vi "Build Bank Engine Group.vi"(8 "error in (no error)":errorcluster, 11 "Device ref dup":T1 format="%.0x") -> (0 "error out":errorcluster, 2 "Group":T2 {"VS Refs" format="%.0x"}, 3 "Section Ref out":T1 format="%.0x")   [LabVIEW 2017, in "NI 272x Resistive Simulation Custom Device Configuration.lvlib"]
uses:
  NI 272x Resistive Simulation Custom Device Configuration.lvlib
  <vilib>/NI Veristand/Custom Device API/Custom Device Item Ref.ctl
  <vilib>/NI Veristand/Custom Device Tools/Custom Device Utility Library/NI VeriStand - Search for Item by Name.vi
  <vilib>/NI VeriStand/Custom Device Tools/Custom Device Utility Library/Custom Device Utility Library.lvlib
  <vilib>/NI VeriStand/Custom Device API/Custom Device API.lvlib
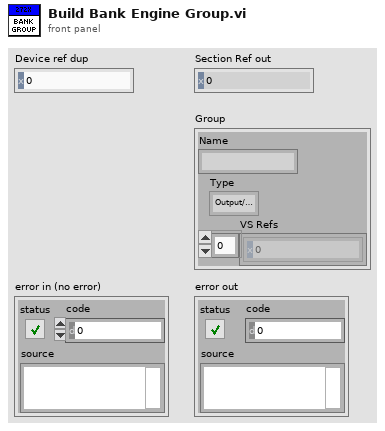
[diagram p1: front panel]
types:
  T1 = typedef "Custom Device API.lvlib/Custom Device Item Ref.ctl" = u64
  T2 = cluster{"Name":string, "Type":enum16{"Output/Write", "Input/Read", "Input/ReadWrite"}, "VS Refs":T1[]}
  T3 = enum16{"Output/Write", "Input/Read", "Input/ReadWrite"}
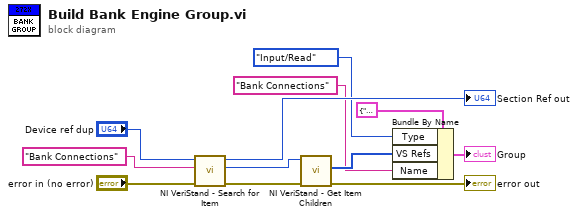
[diagram p0: block diagram]
diagram:
  n1 = call-poly <vilib>:"NI VeriStand - Search for Item.vi"("error in"="error in (no error)", "Item Name"="Bank Connections", "Section Ref in"="Device ref dup") -> ("error out"=w4:errorcluster, "Item Ref"=w6:T1, "Section Ref out"=→"Section Ref out":T1)  [unwired: 5 in, 1 out]
  n2 = call <vilib>:"NI VeriStand - Get Item Children.vi"("error in (no error)"=w4, "Item Ref in"=w6) -> ("error out"=→"error out":errorcluster, "Child Refs"=w12:T1[])  [unwired: 6 in, 2 out]
  n3 = Bundle By Name(cluster=T2 {"Name"="", "Type"=enum."Output/Write", "VS Refs"=[]} ("Group"), "Type"=T3."Input/Read", "VS Refs"=w12, "Name"="Bank Connections" ("Item Name")) -> (→"Group":T2)
